vi "While condition.vi"   [LabVIEW 2019, in "Exaprom PDF.lvlib"]
uses:
  Exaprom PDF.lvlib
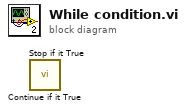
[diagram p0: block diagram]
diagram:
  n1 = call "Continue if it True.vi"() -> ()  [unwired: 7 in, 2 out]
  n2 = call "Stop if it True.vi"() -> ()  [unwired: 7 in, 2 out]
